vi "ex_2_ES_main.vi"() -> ()   [LabVIEW 2020]
uses:
  #typedef_Sound_Intensity.ctl
  <vilib>/Utility/miscctls.llb/LVPositionTypeDef.ctl
  #typedef_ProgramData_ex2.ctl
panel:
  in  "ProgramData":T1={"MousePressed?"=TRUE, "GetKeys"=""}
  in  "Position":T2
  out "To be moved":string
  in  "Sound intensity: MAX":dbl=100.0
  in  "Sound intensity: MIN":dbl
  out "Limit exceeded?":bool
  in  "Stop Button":bool
  in  "Sound intensity [dB]":T3 scale=0.0..100.0
  # "85 dB"
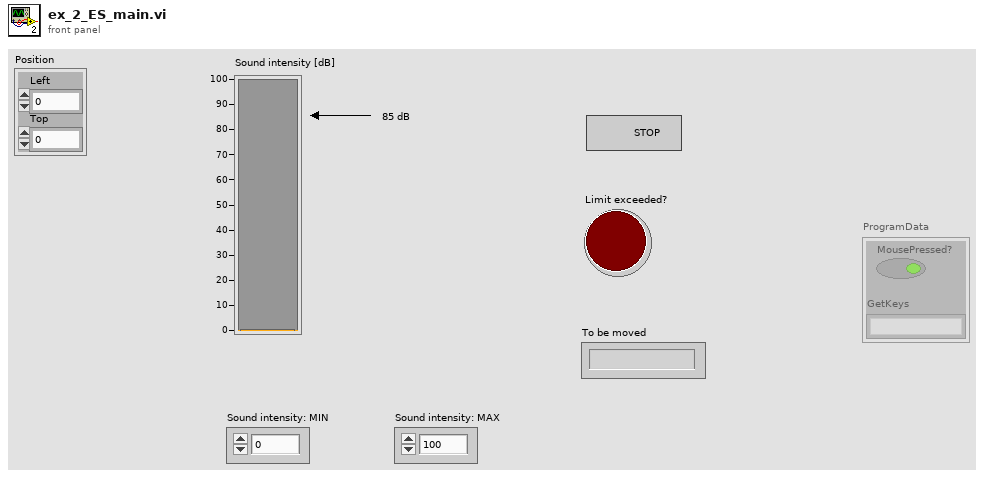
[diagram p1: front panel]
types:
  T1 = typedef "#typedef_ProgramData_ex2.ctl" = cluster{"MousePressed?":bool, "GetKeys":string}
  T2 = typedef "LVPositionTypeDef.ctl" = cluster{"Left":i32, "Top":i32}
  T3 = typedef "#typedef_Sound_Intensity.ctl" = dbl
  T4 = typedef "LVPoint32TypeDef.ctl" = cluster{"Horizontal":i32, "Vertical":i32}
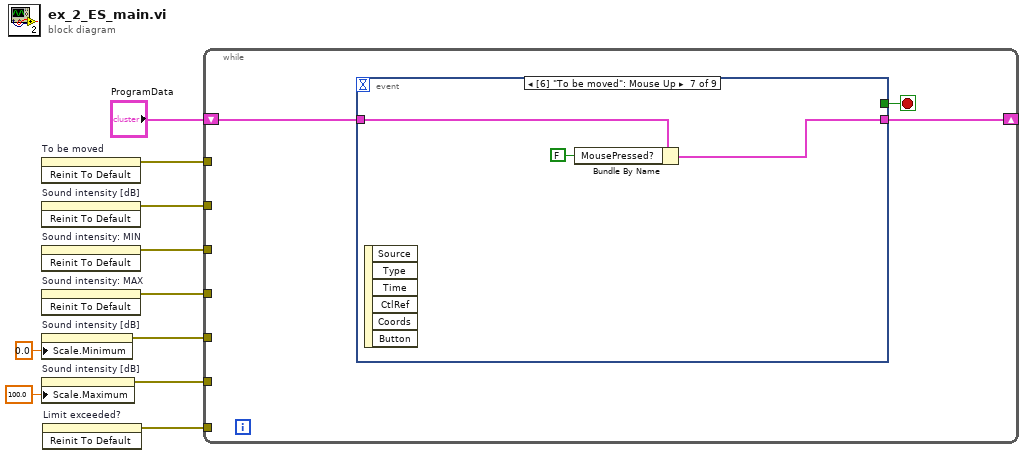
[diagram p0: block diagram]
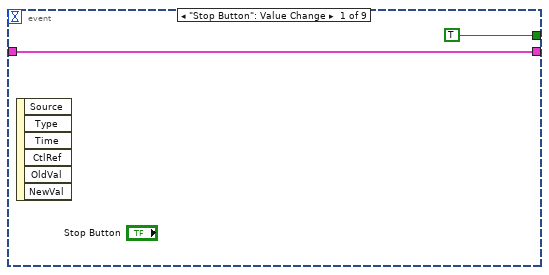
[diagram p2: hidden frame]
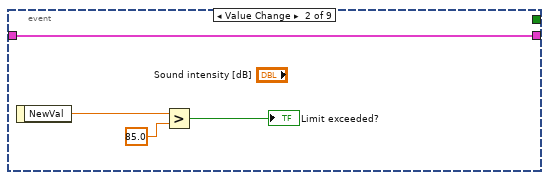
[diagram p3: hidden frame]
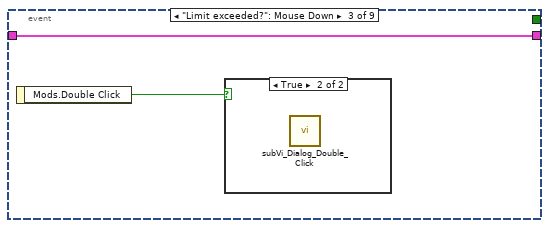
[diagram p4: hidden frame]
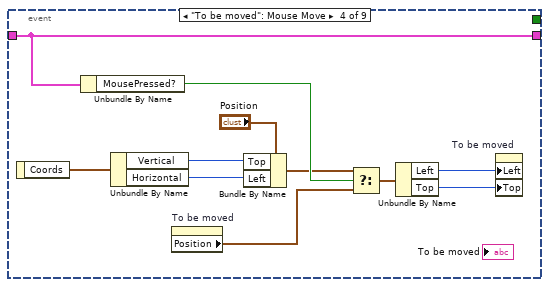
[diagram p6: hidden frame]
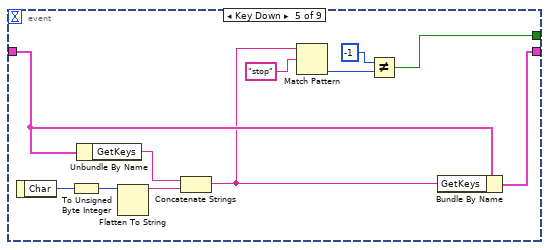
[diagram p7: hidden frame]
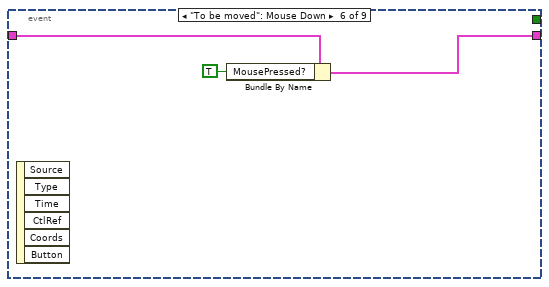
[diagram p8: hidden frame]
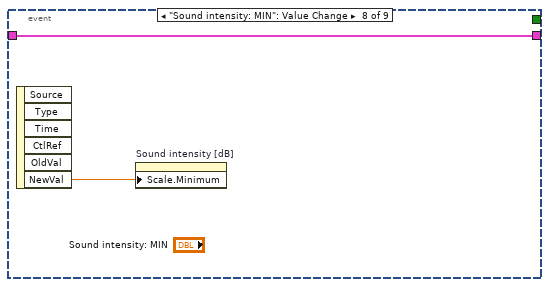
[diagram p9: hidden frame]
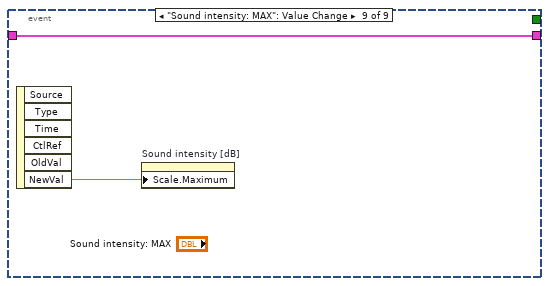
[diagram p10: hidden frame]
diagram:
  n1 = invoke on="To be moved" class="Str" method="Reinit To Default"() -> (error out=w10:errorcluster)  [unwired: 3 in, 2 out]
  n2 = invoke on="Sound intensity [dB]" class="Slide (strict)" method="Reinit To Default"() -> (error out=w9:errorcluster)  [unwired: 3 in, 2 out]
  n3 = invoke on="Sound intensity: MIN" class="DigNum (strict)" method="Reinit To Default"() -> (error out=w8:errorcluster)  [unwired: 3 in, 2 out]
  n4 = invoke on="Sound intensity: MAX" class="DigNum (strict)" method="Reinit To Default"() -> (error out=w7:errorcluster)  [unwired: 3 in, 2 out]
  n5 = property on="Sound intensity [dB]" class="Slide (strict)"("Scale.Minimum"=0.0 ("Scale.Range:Minimum")) -> (error out=w6:errorcluster)  [unwired: 2 in, 1 out]
  n6 = property on="Sound intensity [dB]" class="Slide (strict)"("Scale.Maximum"=100.0 ("Scale.Range:Maximum")) -> (error out=w5:errorcluster)  [unwired: 2 in, 1 out]
  n7 = invoke on="Limit exceeded?" class="Bool (strict)" method="Reinit To Default"() -> (error out=w2:errorcluster)  [unwired: 3 in, 2 out]
  n8 = while {
    shift-right: [w11] -> _
    shift-left: "ProgramData" -> [w12]
    tunnel: w10 -> [_]
    tunnel: w9 -> [_]
    tunnel: w8 -> [_]
    tunnel: w7 -> [_]
    tunnel: w6 -> [_]
    tunnel: w5 -> [_]
    tunnel: w2 -> [_]
    stop <- w13 stop-if-true
    n9 = event shown="[6] \"To be moved\": Mouse Up" {
      selector: _ -> [_ _ _ _ _ _ _ _ _]
      dyn-events: _ -> [_ _ _ _ _ _ _ _ _]
      timeout: _ -> [_ _ _ _ _ _ _ _ _]
      tunnel: [TRUE _ _ _ w33 _ _ _ _] -> w13
      tunnel: [w14 w16 w20 w30 w38 w45 w48 w50 w52] -> w11
      tunnel: w12 -> [w14 w16 w20 w30 w42 w46 w49 w50 w52]
      event "Stop Button": Value Change {
        n10 = event-data() -> ()  [unwired: 1 in, 6 out]
      }
      event Value Change {
        n11 = event-data() -> ("NewVal"=w19:T3)  [unwired: 1 in]
        n12 = Greater?(x=w19, y=85.0) -> (0:→"Limit exceeded?":bool)
      }
      event "Limit exceeded?": Mouse Down {
        n13 = event-data() -> ("Mods.Double Click"=w21:bool)  [unwired: 1 in]
        n14 = case shown="True" w21 {
          frame False {
          }
          frame True {
            n15 = call "subVi_Dialog_Double_Click.vi"() -> ()  [unwired: 12 in]
          }
        }
      }
      event "To be moved": Mouse Move {
        n16 = event-data() -> ("Coords"=w26:T4)  [unwired: 1 in]
        n17 = Unbundle By Name(w30) -> ("MousePressed?"=w28:bool)
        n18 = Unbundle By Name(w26) -> ("Vertical"=w24:i32, "Horizontal"=w23:i32)
        n19 = property on="To be moved" class="Str"() -> ("Position"=w27:T2)  [unwired: 2 in, 2 out]
        n20 = Bundle By Name(cluster="Position", "Top"=w24, "Left"=w23) -> (w22:T2)
        n21 = Select(t=w22, s=w28, f=w27) -> (s? t:f=w29:T2)
        n22 = Unbundle By Name(w29) -> ("Left"=w32:i32, "Top"=w31:i32)
        n23 = property on="To be moved" class="Str"("Left"=w32, "Top"=w31) -> ()  [unwired: 2 in, 2 out]
      }
      event Key Down {
        n24 = event-data() -> ("Char"=w43:i16)  [unwired: 1 in]
        n25 = To Unsigned Byte Integer(number=w43) -> (unsigned 8bit integer=w39:u8)
        n26 = Unbundle By Name(w42) -> ("GetKeys"=w41:string)
        n27 = Flatten To String(anything=w39) -> (data string=w40:string)  [unwired: 3 in, 2 out]
        n28 = Concatenate Strings(w41, w40) -> (w37:string)
        n29 = Match Pattern(string=w37, regular expression="stop") -> (offset past match=w35:i32)  [unwired: 1 in, 3 out]
        n30 = Not Equal?(x=-1, y=w35) -> (x != y?=w33:bool)
        n31 = Bundle By Name(cluster=w42, "GetKeys"=w37) -> (w38:T1)
      }
      event "To be moved": Mouse Down {
        n32 = event-data() -> ()  [unwired: 1 in, 6 out]
        n33 = Bundle By Name(cluster=w46, "MousePressed?"=TRUE) -> (w45:T1)
      }
      event "To be moved": Mouse Up {
        n34 = event-data() -> ()  [unwired: 1 in, 6 out]
        n35 = Bundle By Name(cluster=w49, "MousePressed?"=FALSE) -> (w48:T1)
      }
      event "Sound intensity: MIN": Value Change {
        n36 = event-data() -> ("NewVal"=w51:dbl)  [unwired: 1 in, 5 out]
        n37 = property on="Sound intensity [dB]" class="Slide (strict)"("Scale.Minimum"=w51) -> ()  [unwired: 2 in, 2 out]
      }
      event "Sound intensity: MAX": Value Change {
        n38 = event-data() -> ("NewVal"=w53:dbl)  [unwired: 1 in, 5 out]
        n39 = property on="Sound intensity [dB]" class="Slide (strict)"("Scale.Maximum"=w53) -> ()  [unwired: 2 in, 2 out]
      }
    }
  }
